vi "Event Structure in Empty Space.vi"   [LabVIEW 2017]
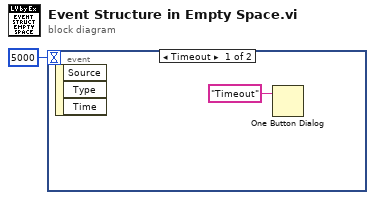
[diagram p0: block diagram]
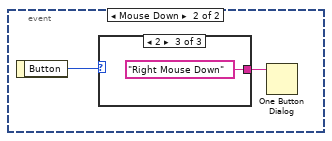
[diagram p2: hidden frame]
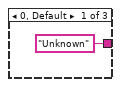
[diagram p3: hidden frame]
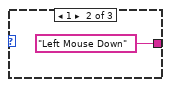
[diagram p4: hidden frame]
diagram:
  n1 = event shown="[0] Timeout" {
    selector: _ -> [_ _]
    dyn-events: _ -> [_ _]
    timeout: 5000 -> [_ _]
    event Timeout {
      n2 = event-data() -> ()  [unwired: 1 in, 3 out]
      n3 = One Button Dialog(message="Timeout") -> ()  [unwired: 1 in, 1 out]
    }
    event Mouse Down {
      n4 = event-data() -> ("Button"=w4:u16)  [unwired: 1 in]
      n5 = case shown="2" w4 {
        tunnel: ["Unknown" "Left Mouse Down" "Right Mouse Down"] -> w3
        frame 0, Default {
        }
        frame 1 {
        }
        frame 2 {
        }
      }
      n6 = One Button Dialog(message=w3) -> ()  [unwired: 1 in, 1 out]
    }
  }
